vi "isMeasureOn.vi"(8 "error in (no error)":errorcluster) -> (0 "error out":errorcluster, 2 "Measure On 2":bool, 3 "Measure On 1":bool)   [LabVIEW 2015, in "ESLSCDLL.lvlib"]
uses:
  ESLSCDLL.lvlib
  Globals.vi
  ESLSCDLL.dll
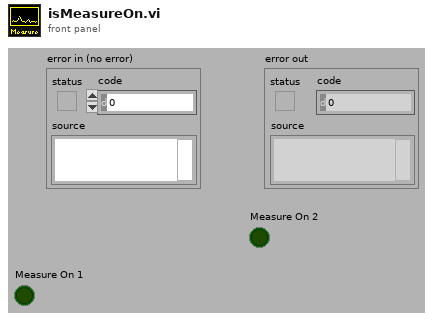
[diagram p1: front panel]
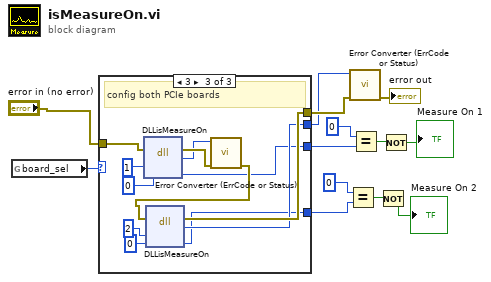
[diagram p0: block diagram]
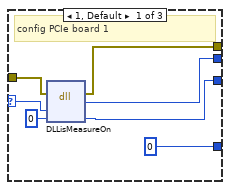
[diagram p2: hidden frame]
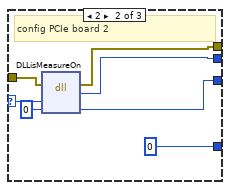
[diagram p3: hidden frame]
diagram:
  n1 = global read "Globals.vi" "board_sel"() -> (w1:u32)
  n2 = case shown="3" w1 {
    selector: w1 -> [w19 w26 _]
    tunnel: [w15 w23 w29] -> w10
    tunnel: [u8 0 ("BlockOn") u8 0 ("BlockOn") w28] -> w7
    tunnel: "error in (no error)" -> [w18 w25 w35]
    tunnel: [w17 w22 w31] -> w3
    tunnel: [w14 w21 w30] -> w2
    frame 1, Default {
      # "config PCIe board 1"
      n3 = dll-call lib="C:/Users/flori/Nextcloud/Dokumente/Stresing/Windows/lv64/board.vis/ESLSCDLL.dll" fn="DLLisMeasureOn" ("lwlscdll.dll:DLLWriteLongS0")(error in=w18, "drv"=w19, "measureOn"=u8 0) -> (error out=w17:errorcluster, "es_status_codes"=w14:i32, "measureOn"=w15:u8)  [unwired: 3 in, 1 out]
    }
    frame 2 {
      # "config PCIe board 2"
      n4 = dll-call lib="C:/Users/flori/Nextcloud/Dokumente/Stresing/Windows/lv64/board.vis/ESLSCDLL.dll" fn="DLLisMeasureOn" ("lwlscdll.dll:DLLWriteLongS0")(error in=w25, "drv"=w26, "measureOn"=u8 0) -> (error out=w22:errorcluster, "es_status_codes"=w21:i32, "measureOn"=w23:u8)  [unwired: 3 in, 1 out]
    }
    frame 3 {
      # "config both PCIe boards"
      n5 = dll-call lib="C:/Users/flori/Nextcloud/Dokumente/Stresing/Windows/lv64/board.vis/ESLSCDLL.dll" fn="DLLisMeasureOn" ("lwlscdll.dll:DLLWriteLongS0")(error in=w35, "drv"=u32 1, "measureOn"=u8 0) -> (error out=w34:errorcluster, "es_status_codes"=w33:i32, "measureOn"=w29:u8)  [unwired: 3 in, 1 out]
      n6 = call "Error Converter (ErrCode or Status).vi"("error in (no error)"=w34, "error code"=w33) -> ("error out"=w32:errorcluster)  [unwired: 9 in]
      n7 = dll-call lib="C:/Users/flori/Nextcloud/Dokumente/Stresing/Windows/lv64/board.vis/ESLSCDLL.dll" fn="DLLisMeasureOn" ("lwlscdll.dll:DLLWriteLongS0")(error in=w32, "drv"=u32 2, "measureOn"=u8 0) -> (error out=w31:errorcluster, "es_status_codes"=w30:i32, "measureOn"=w28:u8)  [unwired: 3 in, 1 out]
    }
  }
  n8 = Equal?(x=u8 0, y=w7) -> (x = y?=w8:bool)
  n9 = call "Error Converter (ErrCode or Status).vi"("error in (no error)"=w3, "error code"=w2) -> ("error out"=→"error out":errorcluster)  [unwired: 9 in]
  n10 = Equal?(x=u8 0, y=w10) -> (x = y?=w12:bool)
  n11 = Not(x=w8) -> (.not. x?=→"Measure On 2":bool)
  n12 = Not(x=w12) -> (.not. x?=→"Measure On 1":bool)
